vi "DeleteStartProcess.vi"(8 "error in (no error)":errorcluster, 11 "AppContextIn":T1={"VIRefToProcessTemplate"=refnum, "VIRefToThisVI"=refnum, "ProcessesList"=[], "VIRefToEnumProcess"=refnum, "VIRefTogetProcessViPath"=refnum, "ProcessManagement"={"EnumProcessState"=enum."Create process", "ProcessName"="", "PathToProcess"=path ""}, "VIRefToSetup"=refnum, "VIRefToStartProcess"=refnum, "ProcessConfig"={"File Path Control"=path "", "Timeout"=0.0, "viInitString"="", "State"=enum."Closed"}}) -> (0 "error out":errorcluster, 3 "AppContextOut":T1={"VIRefToProcessTemplate"=refnum, "VIRefToThisVI"=refnum, "ProcessesList"=[], "VIRefToEnumProcess"=refnum, "VIRefTogetProcessViPath"=refnum, "ProcessManagement"={"EnumProcessState"=enum."Create process", "ProcessName"="", "PathToProcess"=path ""}, "VIRefToSetup"=refnum, "VIRefToStartProcess"=refnum, "ProcessConfig"={"File Path Control"=path "", "Timeout"=0.0, "viInitString"="", "State"=enum."Closed"}})   [LabVIEW 2011]
uses:
  Ctl/AppContext.ctl
  Ctl/EnumProcessState.ctl
  050 - CONFIG/20 - ExternalProcesses/paramsExternalProcesses.ctl
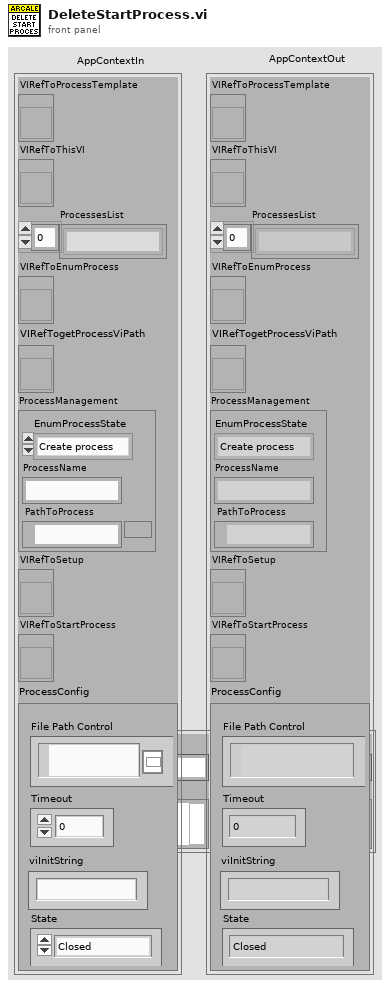
[diagram p1: front panel]
types:
  T1 = typedef "AppContext.ctl" = cluster{"VIRefToProcessTemplate":refnum<vi>, "VIRefToThisVI":refnum<vi>, "ProcessesList":string[], "VIRefToEnumProcess":refnum<vi>, "VIRefTogetProcessViPath":refnum<vi>, "ProcessManagement":cluster{"EnumProcessState":T2, "ProcessName":string, "PathToProcess":path}, "VIRefToSetup":refnum<vi>, "VIRefToStartProcess":refnum<vi>, "ProcessConfig":T3}
  T2 = typedef "EnumProcessState.ctl" = enum16{"Create process", "Delete process"}
  T3 = typedef "paramsExternalProcesses.ctl" = cluster{"File Path Control":path, "Timeout":dbl, "viInitString":string, "State":enum32{"Invalid", "Standard", "Closed", "Hidden", "Minimized", "Maximized"}}
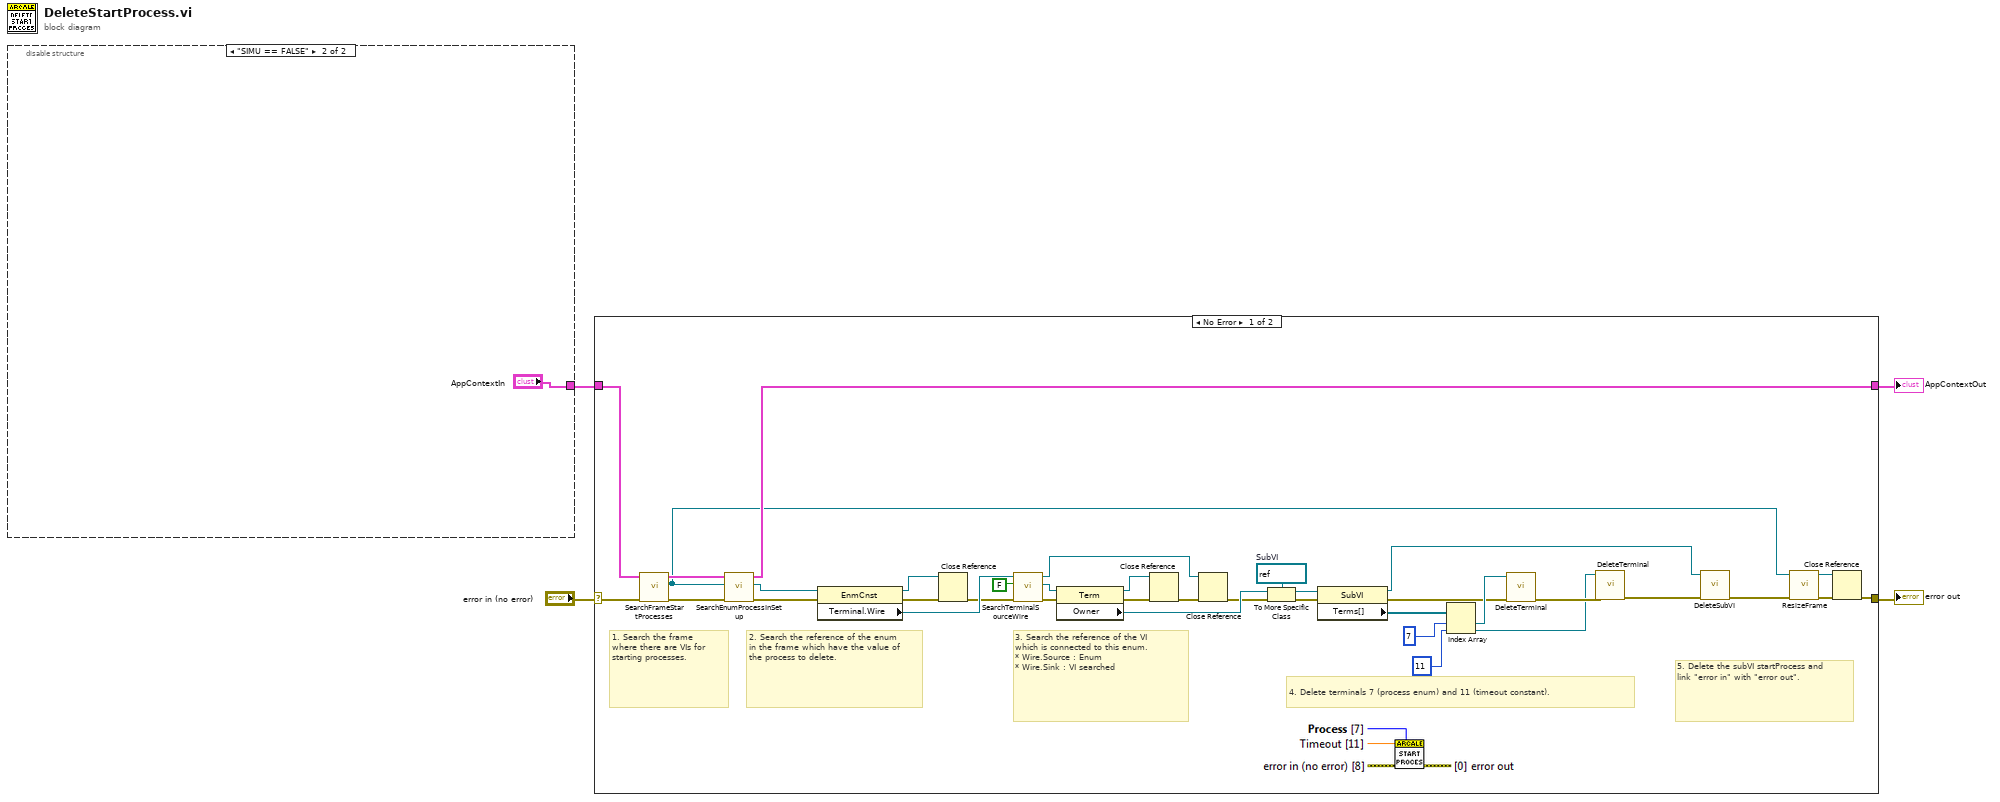
[diagram p0: block diagram]
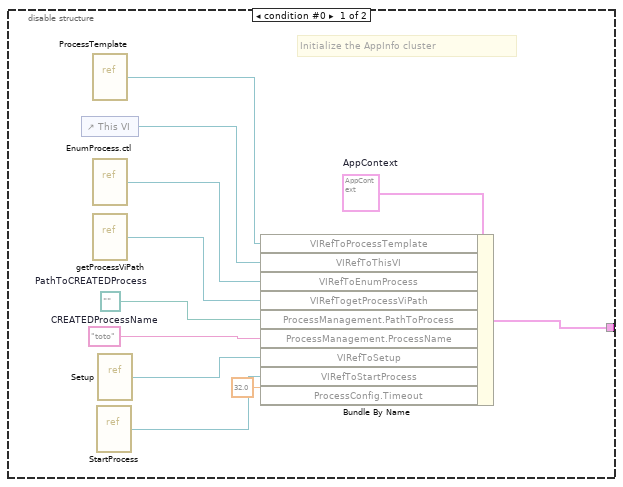
[diagram p2: hidden frame]
diagram:
  n1 = disable-structure shown="\"SIMU == FALSE\"" {
    disable-tunnel: [w6 "AppContextIn"] -> w1
    frame condition #0 {
      w9 = T1 {"VIRefToProcessTemplate"=refnum, "VIRefToThisVI"=refnum, "ProcessesList"=[], "VIRefToEnumProcess"=refnum, "VIRefTogetProcessViPath"=refnum, "ProcessManagement"={"EnumProcessState"=enum."Create process", "ProcessName"="", "PathToProcess"=path ""}, "VIRefToSetup"=refnum, "VIRefToStartProcess"=refnum, "ProcessConfig"={"File Path Control"=path "", "Timeout"=0.0, "viInitString"="", "State"=enum."Invalid"}}  # AppContext
      w10 = "toto"  # CREATEDProcessName
      w11 = path ""  # PathToCREATEDProcess
      # "Initialize the AppInfo cluster"
      n2 = control-ref of="This VI"() -> (w14:refnum<vi>)
      n3 = vi-ref "ProcessTemplate.vi"() -> (w15:refnum<vi>)
      n4 = vi-ref "EnumProcess.ctl"() -> (w13:refnum<vi>)
      n5 = vi-ref "getProcessViPath.vi"() -> (w12:refnum<vi>)
      n6 = vi-ref "StartProcess.vi"() -> (w7:refnum<vi>)
      n7 = vi-ref "Setup.vi"() -> (w8:refnum<vi>)
      n8 = Bundle By Name(cluster=w9, "VIRefToProcessTemplate"=w15, "VIRefToThisVI"=w14, "VIRefToEnumProcess"=w13, "VIRefTogetProcessViPath"=w12, "ProcessManagement.PathToProcess"=w11, "ProcessManagement.ProcessName"=w10, "VIRefToSetup"=w8, "VIRefToStartProcess"=w7, "ProcessConfig.Timeout"=32.0 ("ProcessManagement.Timeout")) -> (w6:T1)
    }
    frame condition #1 (active) {
    }
  }
  n9 = case shown="No Error" "error in (no error)" {
    selector: "error in (no error)" -> [w53 w55]
    tunnel: [w17 w55] -> w3
    tunnel: [w47 w54] -> w2
    tunnel: w1 -> [w50 w54]
    frame No Error {
      w45 = refnum<vi> refnum  # SubVI
      # "5. Delete the subVI startProcess and link \"error in\" with \"error out\"."
      # "4. Delete terminals 7 (process enum) and 11 (timeout constant)."
      # "3. Search the reference of the VI which is connected to this enum.\n* Wire.Source : Enum\n* Wire.Sink : VI searched"
      # "2. Search the reference of the enum in the frame which have the value of the process to delete."
      # "1. Search the frame where there are VIs for starting processes."
      n10 = call "SearchFrameStartProcesses.vi"("error in (no error)"=w53, "AppContextIn"=w50) -> ("error out"=w52:errorcluster, "FlatSequenceFrame out"=w20:refnum<vi>, "AppContextOut"=w49:T1)  [unwired: 7 in]
      n11 = call "SearchEnumProcessInSetup.vi"("error in (no error)"=w52, "FlatSequenceFrame in"=w20, "AppContextIn"=w49) -> ("error out"=w51:errorcluster, "EnumConstant out"=w48:refnum<vi>, "AppContextOut"=w47:T1)  [unwired: 6 in]
      n12 = property class="EnmCnst"(reference=w48, error in=w51) -> (reference out=w27:refnum<vi>, error out=w29:errorcluster, "Terminal.Wire"=w43:refnum<vi>)
      n13 = Close Reference(reference=w27, error in (no error)=w29) -> (error out=w28:errorcluster)
      n14 = call "SearchTerminalSourceWire.vi"("error in (no error)"=w28, "Source?"=FALSE, "Refnum Wire In"=w43) -> ("error out"=w44:errorcluster, "Terminal Refnum"=w41:refnum<vi>, "Refnum Wire Out"=w24:refnum<vi>)  [unwired: 6 in]
      n15 = property class="Term"(reference=w41, error in=w44) -> (reference out=w26:refnum<vi>, error out=w23:errorcluster, "Owner"=w46:refnum<vi>)
      n16 = Close Reference(reference=w26, error in (no error)=w23) -> (error out=w25:errorcluster)
      n17 = Close Reference(reference=w24, error in (no error)=w25) -> (error out=w22:errorcluster)
      n18 = To More Specific Class(target class=w45, reference=w46, error in=w22) -> (specific class reference=w32:refnum<vi>, error out=w33:errorcluster)
      n19 = property class="SubVI"(reference=w32, error in=w33) -> (reference out=w31:refnum<vi>, error out=w35:errorcluster, "Terms[]"=w38:refnum<vi>[])
      n20 = Index Array(array=w38, index #1=7 ("index"), index #2=11 ("index")) -> (element #1=w39:refnum<vi>, element #2=w30:refnum<vi>)
      n21 = call "DeleteTerminal.vi"("error in (no error)"=w35, "Refnum TerminalToDelete"=w39) -> ("error out"=w40:errorcluster)  [unwired: 9 in]
      n22 = call "DeleteTerminal.vi"("error in (no error)"=w40, "Refnum TerminalToDelete"=w30) -> ("error out"=w34:errorcluster)  [unwired: 9 in]
      n23 = call "DeleteSubVI.vi"("error in (no error)"=w34, "SubVI in"=w31) -> ("error out"=w21:errorcluster)  [unwired: 9 in]
      n24 = call "ResizeFrame.vi"("error in (no error)"=w21, "FlatSequenceFrame in"=w20) -> ("error out"=w18:errorcluster, "FlatSequenceFrame out"=w19:refnum<vi>)  [unwired: 8 in]
      n25 = Close Reference(reference=w19, error in (no error)=w18) -> (error out=w17:errorcluster)
    }
    frame Error {
    }
  }
  "error out" <- w3
  "AppContextOut" <- w2
